vi "Bind Listbox Item Names.vi"(8 "error in (no error)":errorcluster, 9 "Datum Name (\"\"=Use Control Label)":string, 10 "LstBox Refnum":refnum<vi>, 11 "IViewable in":refnum<class "IViewable.lvclass">) -> (0 "error out":errorcluster, 3 "IViewable out":refnum<class "IViewable.lvclass">)   [LabVIEW 2018, in "MVA Framework.lvlib" / "IViewable.lvlib" / "IViewable.lvclass"]
doc: "将单列列表框的项目名称绑定到已发布的1-D字符串数组。"
uses:
  IViewable.lvclass
  mva-core/Source/IMediator/SubscriptionRequest/SubscriptionRequest.lvclass
  mva-core/Source/IObserver/IObserver Messages/Subscribe Msg/Subscribe Msg.lvclass
  <vilib>/ActorFramework/Actor/Actor.lvclass
  mva-core/Source/IMediator/ISubscriptionPolicy/ISubscriptionPolicy.lvclass
  mva-core/Source/SubscriptionPolicy/ValueChangeSubscription/ValueChangeSubscription.lvclass
  composed-transport/Source/Concrete/ListboxItemNamesBinding/ListboxItemNamesBinding.lvclass
  C:/Program Files/National Instruments/LabVIEW 2020/vi.lib/ActorFramework/Actor/Actor.lvclass
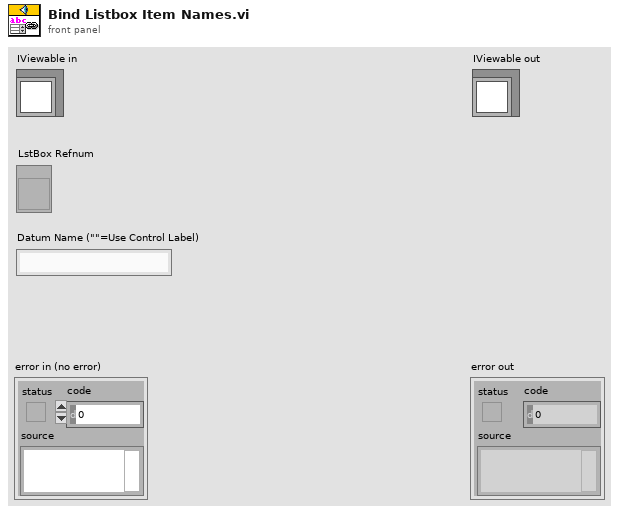
[diagram p1: front panel]
types:
  T1 = typedef "MVA Framework.lvlib/IMediator.lvlib/ISubscriptionPolicy.lvclass/ISubscriptionPolicy Reference.ctl" = refnum<data-value>
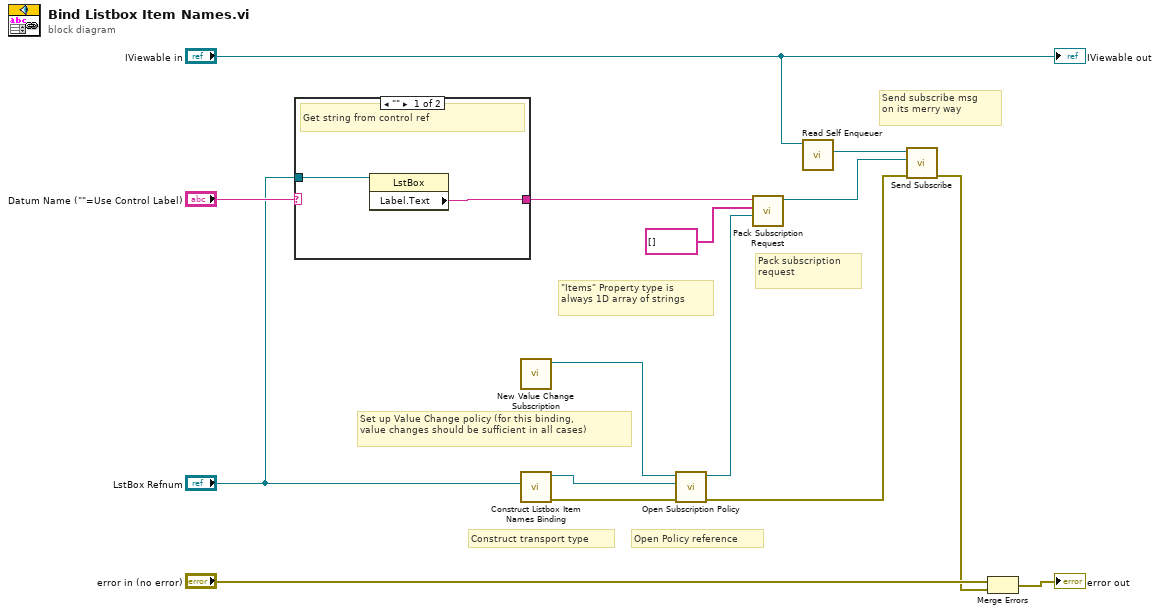
[diagram p0: block diagram]
diagram:
  # "\"Items\" Property type is\nalways 1D array of strings"
  # "Open Policy reference"
  # "Set up Value Change policy (for this binding,\nvalue changes should be sufficient in all cases)"
  # "Send subscribe msg\non its merry way"
  # "Pack subscription\nrequest"
  # "Construct transport type"
  n1 = case shown="\"\"" "Datum Name (\"\"=Use Control Label)" {
    selector: "Datum Name (\"\"=Use Control Label)" -> [_ w18]
    tunnel: [w16 w18] -> w9
    tunnel: "LstBox Refnum" -> [w17 _]
    frame "" {
      # "Get string from control ref"
      n2 = property class="LstBox"(reference=w17) -> ("Label.Text"=w16:string)  [unwired: 1 in, 2 out]
    }
    frame Default {
      # "Use string wired to input terminal"
    }
  }
  n3 = call "New Value Change Subscription.vi"() -> ("ValueChangeSubscription Out"=w5:refnum<class "ValueChangeSubscription.lvclass">)  [unwired: 11 in]
  n4 = call "Construct Listbox Item Names Binding.vi"("LstBox Refnum"="LstBox Refnum") -> ("error out"=w4:errorcluster, "ListboxItemNamesBinding"=w7:refnum<class "ListboxItemNamesBinding.lvclass">)  [unwired: 9 in]
  n5 = call "Open Subscription Policy.vi"("error in (no error)"=w4, "Transport"=w7, "SubscriptionPolicy"=w5) -> ("error out"=w1:errorcluster, "Subscription Policy"=w2:T1)  [unwired: 7 in]
  n6 = call "Pack Subscription Request.vi"("Subscription Policy"=w2, "Type"=string[] [], "Datum Name"=w9) -> ("SubscriptionRequest"=w6:refnum<class "SubscriptionRequest.lvclass">)  [unwired: 7 in, 1 out]
  n7 = call <vilib>:"Read Self Enqueuer.vi"("Actor"="IViewable in") -> ("Self Enqueuer"=w13:refnum<class "Message Enqueuer.lvclass">)  [unwired: 10 in]
  n8 = call "Send Subscribe.vi"("error in (no error)"=w1, "SubscriptionRequest"=w6, "Message Enqueuer"=w13) -> ("error out"=w11:errorcluster)  [unwired: 7 in, 1 out]
  n9 = Merge Errors("error in (no error)", w11) -> (→"error out":errorcluster)
  "IViewable out" <- "IViewable in"
